vi "fpga_transmission_control_3V14.vi"() -> ()   [LabVIEW 2017]
uses:
  Control 1.ctl
  <vilib>/Platform/TimedLoop/XDataNode/timing_clust.ctl
  <vilib>/Platform/TimedLoop/XDataNode/nitl_modes.ctl
  <vilib>/Platform/TimedLoop/XDataNode/wakeup.ctl
  <vilib>/Instr/_visa.llb/VISA Configure Serial Port (Serial Instr).vi
  <vilib>/platform/TimedLoop/XDataNode/XDataNode.xnode
  <vilib>/Platform/TimedLoop/XDataNode/XDNodeRunTimeDep.lvlib
panel:
  out "Complete Time":u32
  out "Timer":u32
  out "Output":bool
  out "outcome":u32
  out "currentType":string
  out "Time":dbl(slide) scale=0.0..100.0
  out "Progress":dbl(slide) scale=0.0..100.0
  in  "error in (no error)":errorcluster
  out "PWM":bool
  out "pattern":u32
  in  "Timeslot":bool
  out "type":string
  out "Kombi Chart":cluster{u16, i16}(graph)
  out "contingency":string
  in  "Array":T2(array[cluster]) {"duration" step=1}
  out "Timeslot":i32
  out "Sign":bool
  out "deleted portion":u8[](array[numeric])
  out "data":bool
  out "x-y":u16
  out "Error String":string
  out "error out":errorcluster
  out "Int_pixel":i16
  out "Pixel":u16(graph)
  out "AD_Value":i16
  in  "millisecond timer value 2":u32
  out "AD_Chart":i16(graph)
  in  "Path":path
  out "Read":bool
  in  "Stop Program":bool
  in  "Start":bool
  in  "VISA resource name":refnum<visa-resource-name>
  # "UR Elektronik Biologie\nTerminal V 3.8"
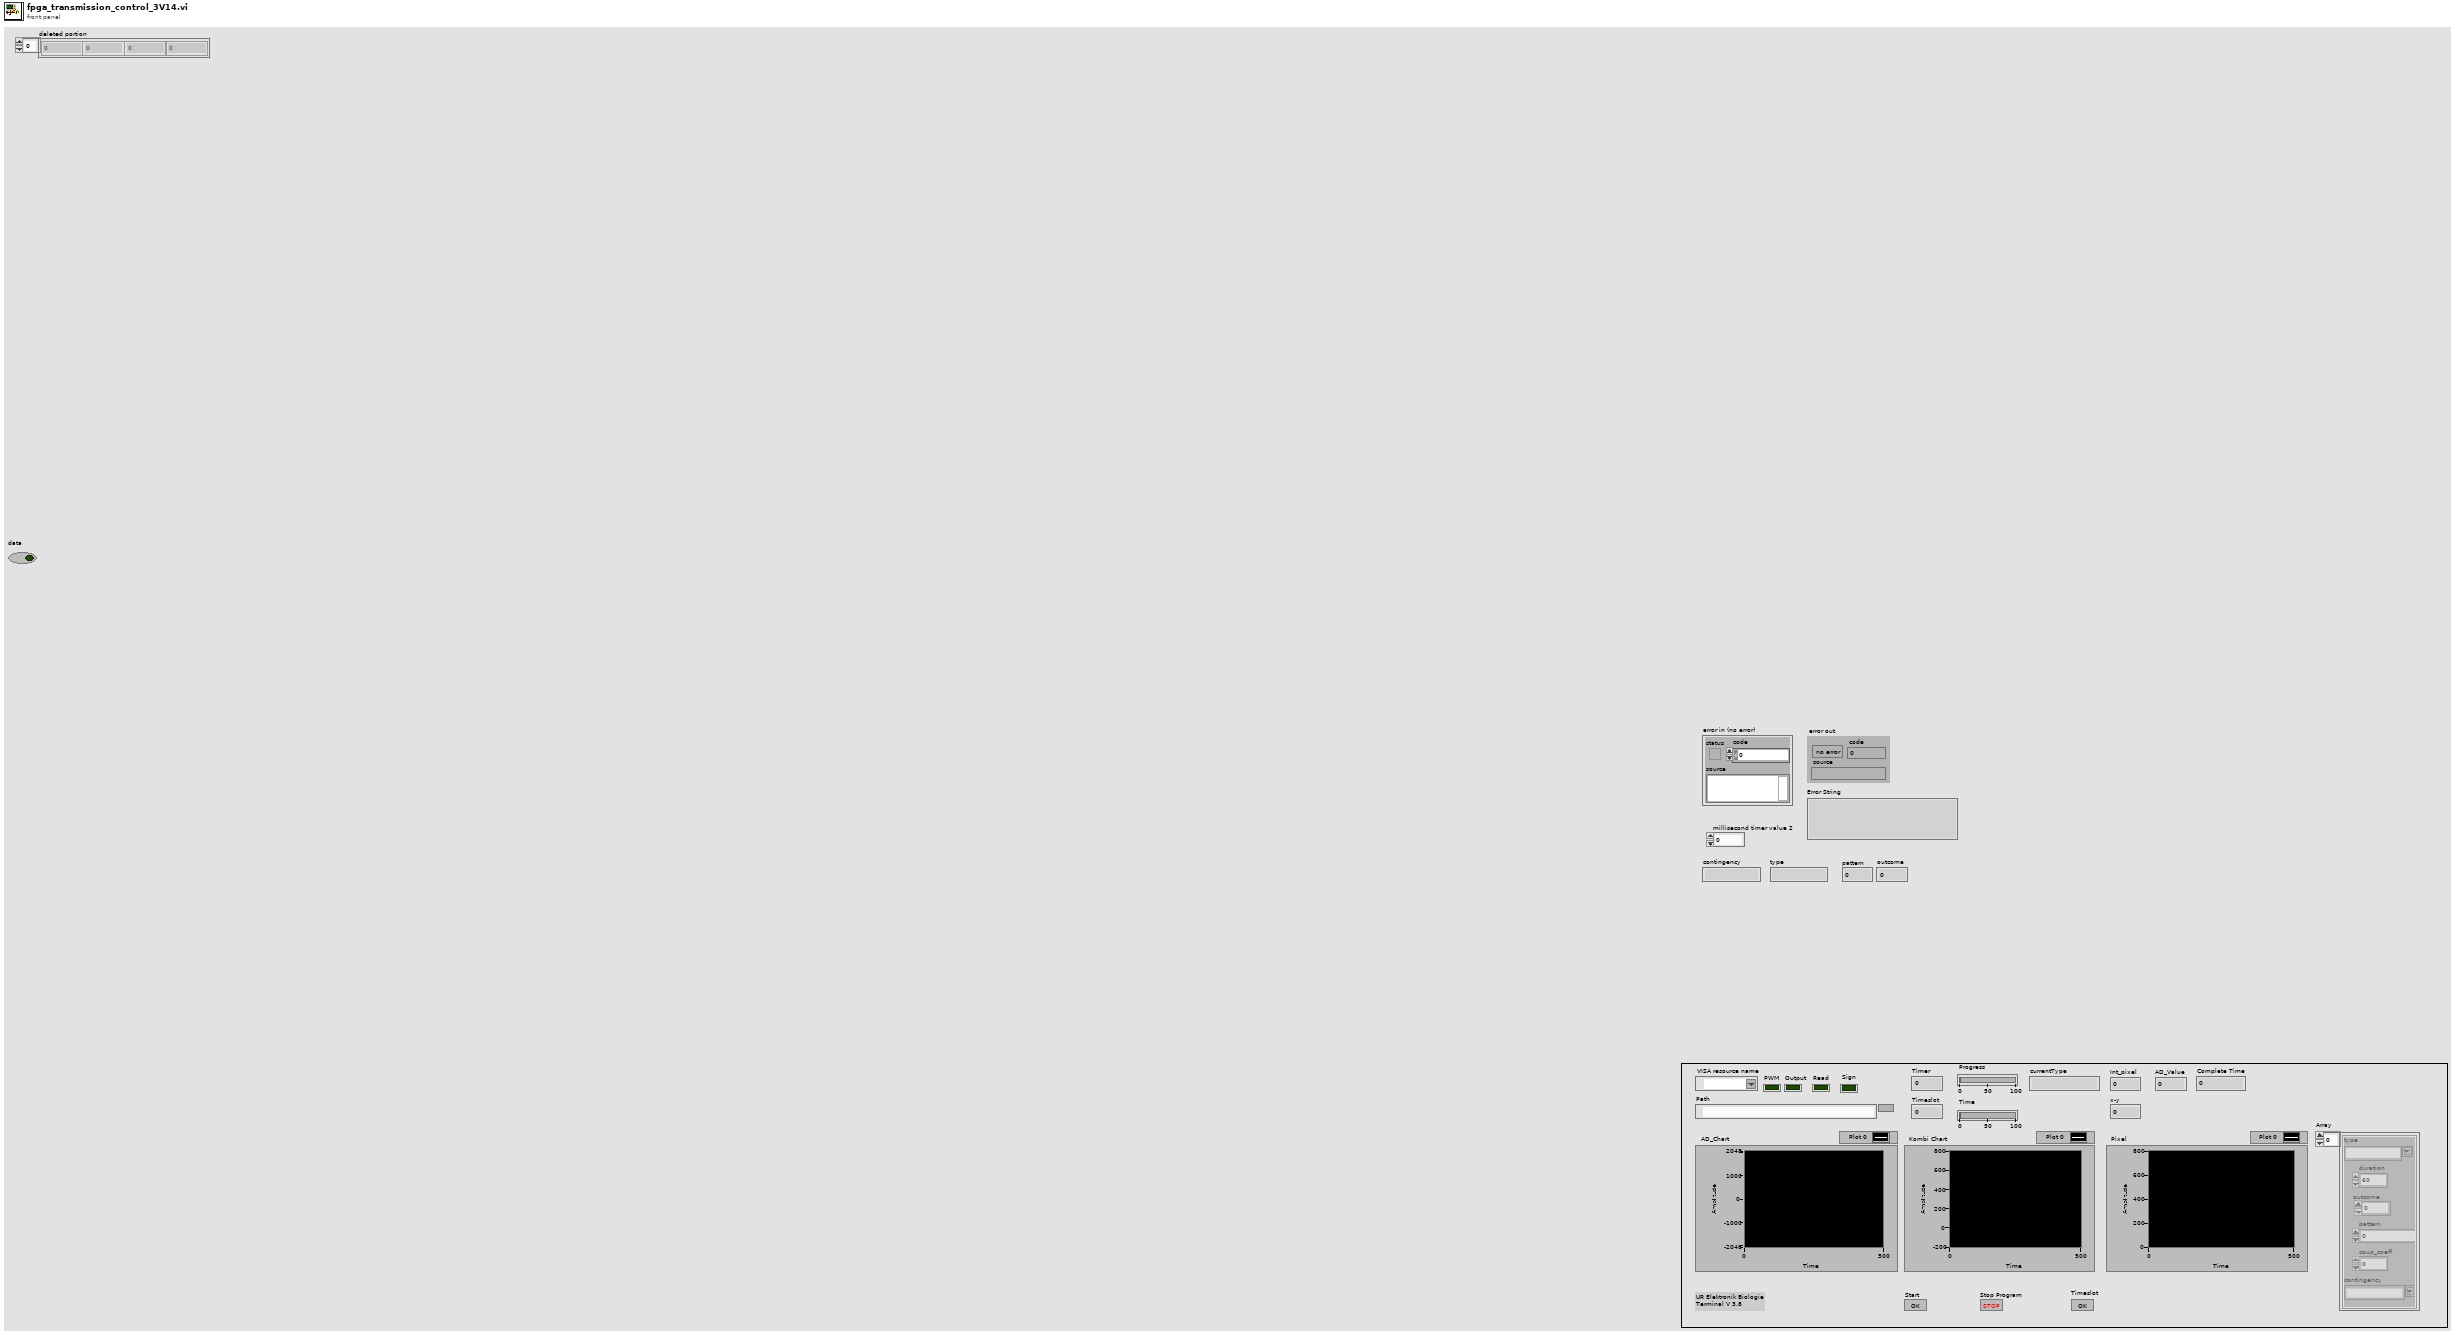
[diagram p1: front panel]
types:
  T1 = typedef "Control 1.ctl" = u32
  T2 = cluster{"type":string, "duration":T1, "outcome":u32, "pattern":u32, "coup_coeff":u32, "contingency":string}[]
  T3 = typedef "XDNodeRunTimeDep.lvlib/timing_clust.ctl" = cluster{"Expected End [f-1]":u64, "Actual End [f-1]":u64, "Finished Late? [f-1]":bool, "Expected End [i-1]":u64, "Actual End [i-1]":u64, "Finished Late? [i-1]":bool, "Expected Start [i]":u64, "Actual Start [i]":u64, "Expected Start [f]":u64, "Actual Start [f]":u64, "Source Name":string, "Structure Name":string, "Period":i64, "Deadline":i64, "Offset":i64, "Start":i64, "Priority":i32, "Timeout":i32, "Mode":T4, "Wakeup Reason":T5, "Error":errorcluster, "Source Type":string, "Secondary Source Type":string, "Global End Time":u64, "Global Start Time":u64, "Frame Duration":u64, "Iteration Duration":u64, "Assigned CPU":i32, "I/O Scan Engine Mode":u32}
  T4 = typedef "XDNodeRunTimeDep.lvlib/nitl_modes.ctl" = enum32{"No Change", "Process missed periods, maintain original phase", "Discard missed periods, maintain original phase", "Process missed periods, ignore original phase", "Discard missed periods, ignore original phase"}
  T5 = typedef "XDNodeRunTimeDep.lvlib/wakeup.ctl" = enum32{"Normal", "Aborted", "Asynchronous wakeup", "Timing source error", "Timed loop error", "Timeout"}
  T6 = cluster{"String":string, i32, i32, u32, u32, "String":string}[]
  T7 = cluster{"type":string, "duration":T1, "outcome":u32, "pattern":u32, "coup_coeff":u32, "contingency":string}
  T8 = enum16{"Idel", "State1", "State2", "State3", "State4"}
  T9 = enum16{"open", "replace", "create", "open or create", "replace or create", "replace or create with confirmation"}
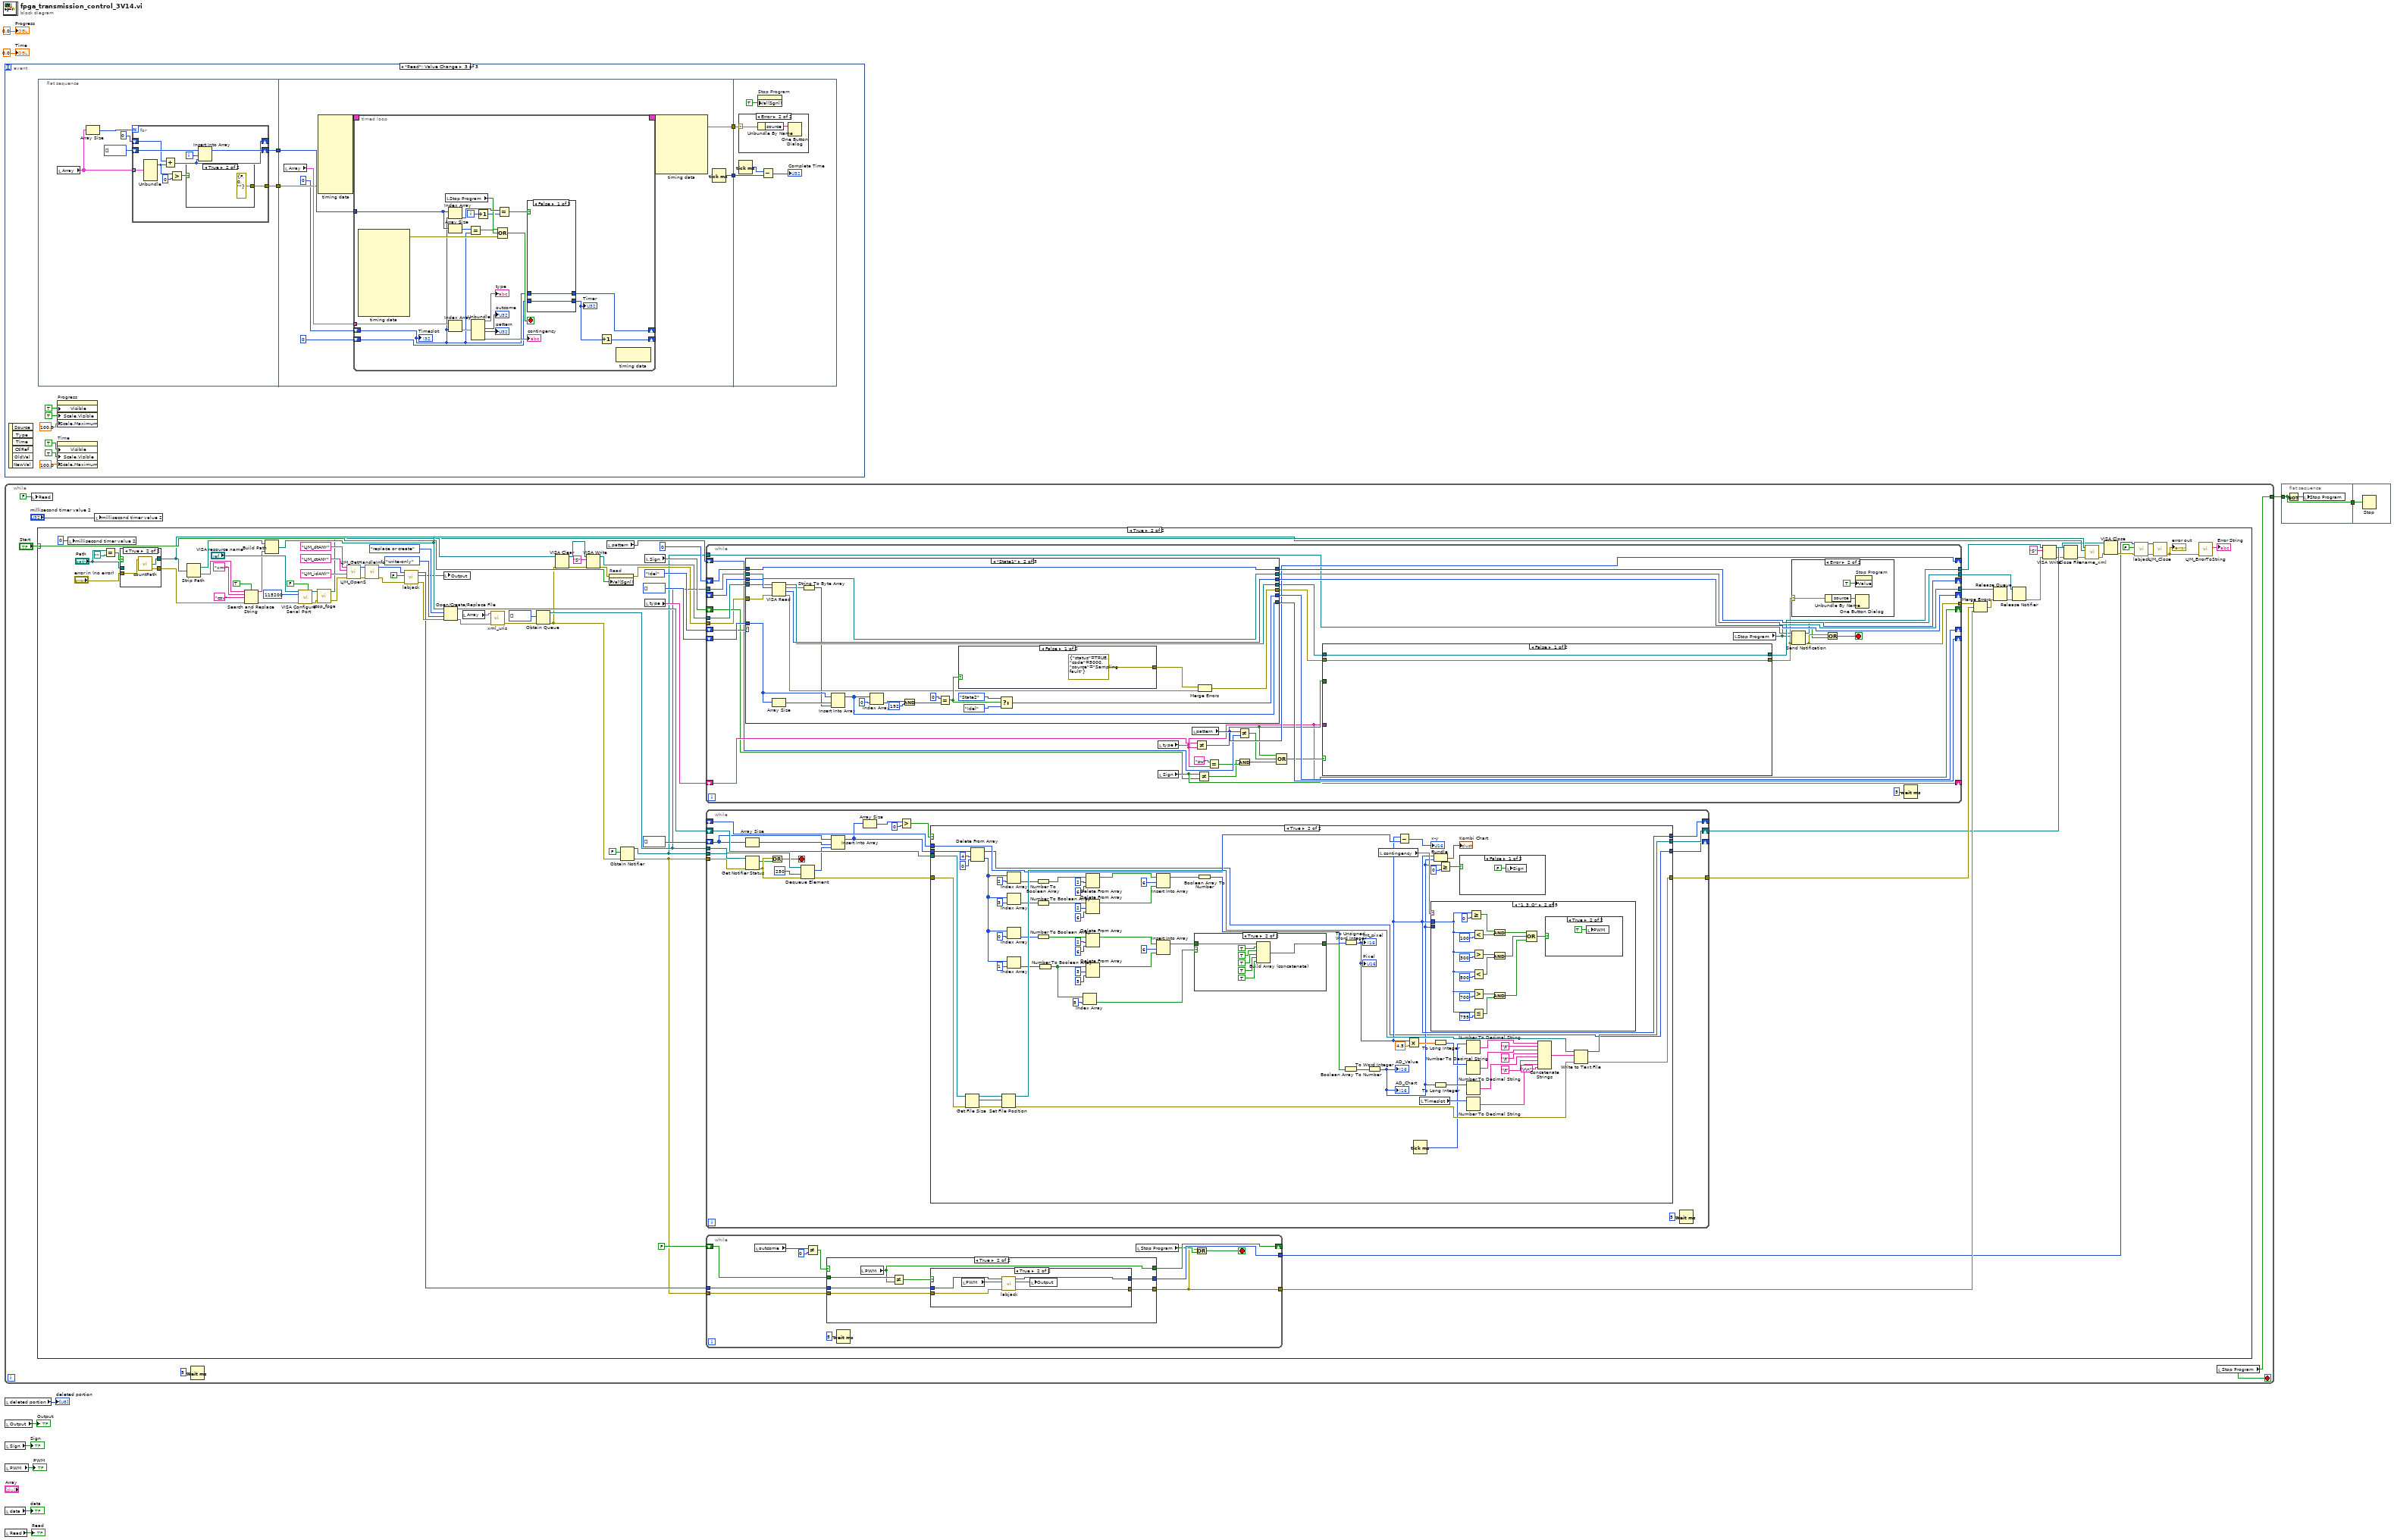
[diagram p0: block diagram]
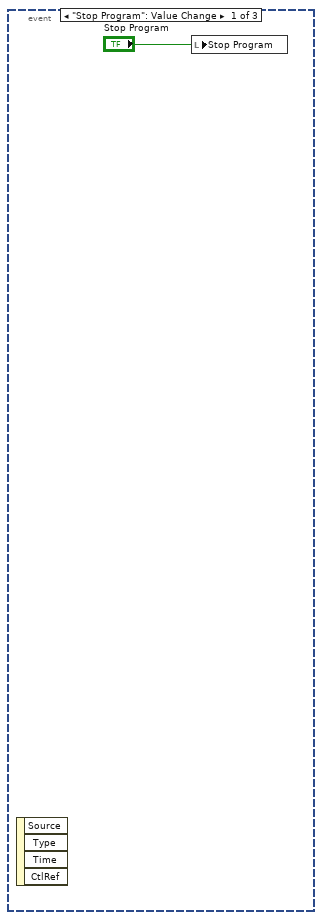
[diagram p2: hidden frame]
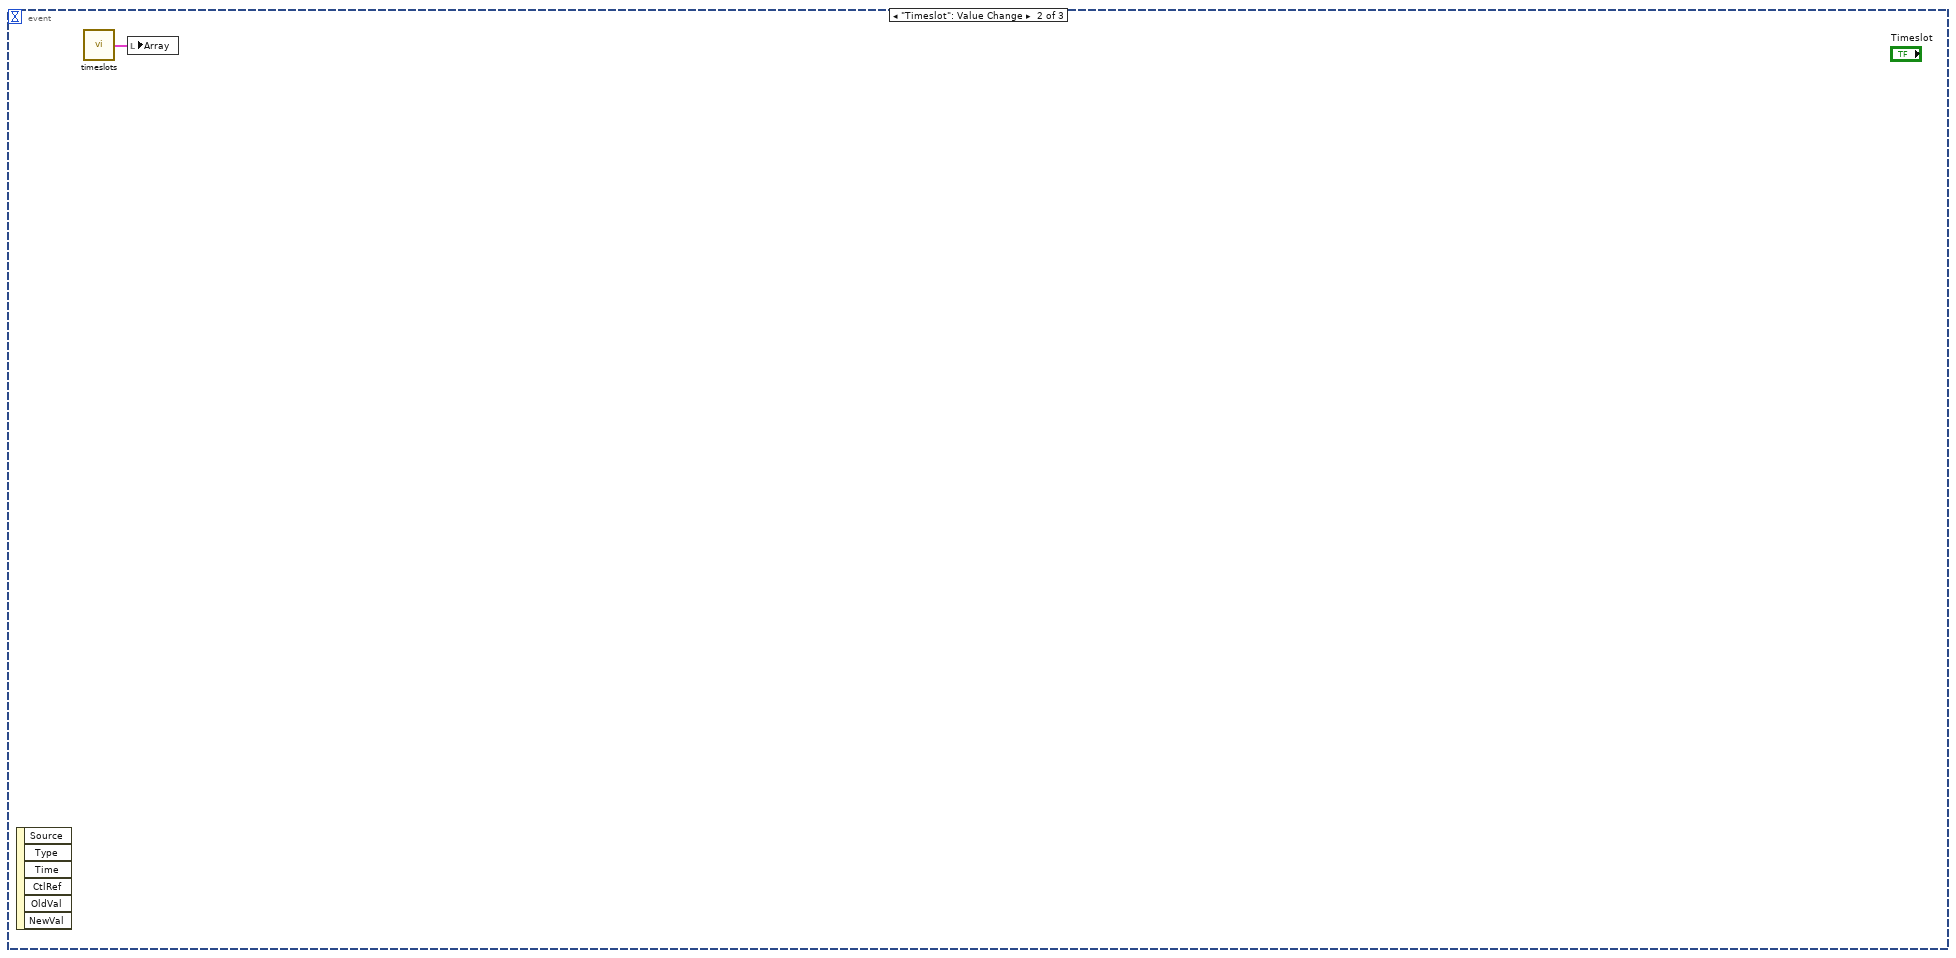
[diagram p3: hidden frame]
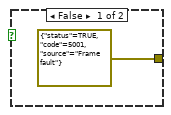
[diagram p4: hidden frame]
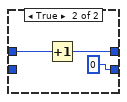
[diagram p5: hidden frame]
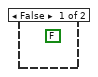
[diagram p7: hidden frame]
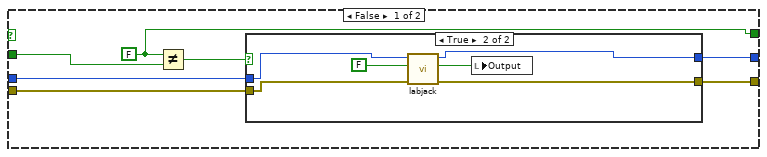
[diagram p9: hidden frame]
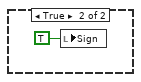
[diagram p13: hidden frame]
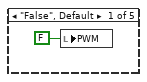
[diagram p14: hidden frame]
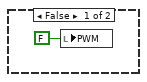
[diagram p15: hidden frame]
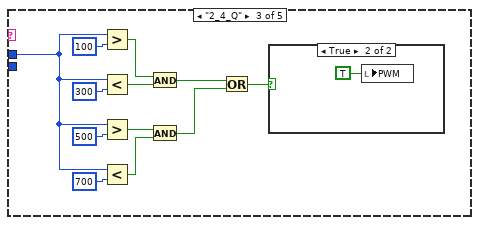
[diagram p16: hidden frame]
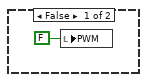
[diagram p17: hidden frame]
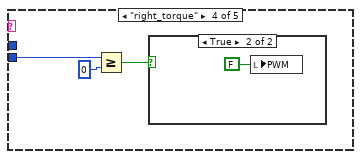
[diagram p18: hidden frame]
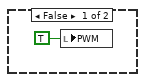
[diagram p19: hidden frame]
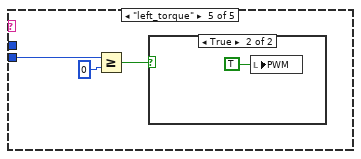
[diagram p20: hidden frame]
diagram:
  n1 = event shown="[2] \"Read\": Value Change" {
    selector: _ -> [_ _ _]
    dyn-events: _ -> [_ _ _]
    timeout: _ -> [_ _ _]
    event "Stop Program": Value Change {
      n2 = event-data() -> ()  [unwired: 1 in, 4 out]
      n3 = local write "Stop Program"("Stop Program") -> ()
    }
    event "Timeslot": Value Change {
      n4 = event-data() -> ()  [unwired: 1 in, 6 out]
      n5 = call "timeslots.vi"() -> ("array of clusters"=w12:T6)  [unwired: 1 in, 1 out]
      n6 = local write "Array"(w12) -> ()
    }
    event "Read": Value Change {
      n7 = event-data() -> ()  [unwired: 1 in, 6 out]
      n8 = flat-sequence {
        tunnel: [w24] -> w16
        tunnel: [w23] -> w15
        tunnel: w16 -> [w46]
        tunnel: w15 -> [w45]
        tunnel: [w44] -> w14
        tunnel: [w42] -> w13
        tunnel: w14 -> [w87]
        tunnel: w13 -> [w84]
        frame #0 {
          n9 = local read "Array"() -> (w27:T2)
          n10 = Array Size(array=w27) -> (size(s)=w28:i32)
          n11 = for {
            N: w28 -> [_]
            tunnel: w27 -> [w38] mode=indexing
            shift-right: [w36] -> w24
            shift-left: T1[] [] -> [w35]
            shift-right: [w33] -> _
            shift-left: T1 0 ("duration") -> [w34]
            tunnel: [w29] -> w23
            i -> [w37]
            n12 = Unbundle(w38) -> ("duration"=w31:T1)  [unwired: 5 out]
            n13 = Add(x=w34, y=w31) -> (x+y=w33:T1)
            n14 = Greater?(x=w31, y=T1 0) -> (0:w32:bool)
            n15 = case shown="True" w32 {
              tunnel: [errorcluster {"status"=TRUE, "code"=5001, "source"="Frame fault"} ("error constant") errorcluster {"status"=FALSE, "code"=0, "source"=""} ("error constant")] -> w29
              frame False {
              }
              frame True {
              }
            }
            n16 = Insert Into Array(array=w35, index=w37, new element=w33) -> (w36:T1[])
          }
        }
        frame #1 {
          n17 = local read "Array"() -> (w47:T2)
          n18 = node-c288(w45) -> (w49:T3)  [unwired: 9 in]
          n19 = timed-loop {
            timing: w49 -> [_]
            timing-out: [_] -> w48
            tunnel: w47 -> [w65]
            tunnel: w46 -> [w59]
            shift-right: [w62] -> _
            shift-left: T1 0 ("duration") -> [w57]
            shift-right: [w52] -> _
            shift-left: 0 -> [w51]
            i -> [w54]
            stop <- w64 stop-if-true
            n20 = node-c288() -> (w63:errorcluster)  [unwired: 1 in, 11 out]
            n21 = local read "Stop Program"() -> (w56:bool)
            n22 = Index Array(array=w59, index=w57) -> (element=w61:T1)
            n23 = Array Size(array=w59) -> (size(s)=w58:i32)
            n24 = Index Array(array=w65, index=w57) -> (element=w70:T7)
            n25 = Equal?(x=w58, y=w57) -> (x = y?=w55:bool)
            n26 = Unbundle(w70) -> ("type"=→"type":string, "outcome"=→"outcome":u32, "pattern"=→"pattern":u32, "contingency"=→"contingency":string)  [unwired: 2 out]
            n27 = Increment(x=w54) -> (x+1=w53:i32)
            n28 = Equal?(x=w61, y=w53) -> (x = y?=w60:bool)
            n29 = Compound Arithmetic op=OR(w56, w55, w63) -> (w64:bool)
            n30 = case shown="False" w60 {
              tunnel: [w72 w75] -> w62
              tunnel: w57 -> [w72 w74]
              tunnel: w51 -> [w71 _]
              tunnel: [w71 0] -> w50
              frame False {
              }
              frame True {
                n31 = Increment(x=w74) -> (x+1=w75:T1)
              }
            }
            "Timer" <- w50
            n32 = Increment(x=w50) -> (x+1=w52:i32)
            n33 = node-c288() -> ()  [unwired: 1 in, 1 out]
            "Timeslot" <- w57
          }
          n34 = node-c288(w48) -> (w44:errorcluster)  [unwired: 6 out]
          n35 = Tick Count (ms)() -> (millisecond timer value=w42:u32)
        }
        frame #2 {
          n36 = case shown="Error" w87 {
            selector: w87 -> [_ w90]
            frame No Error {
            }
            frame Error {
              n37 = Unbundle By Name(w90) -> ("source"=w89:string)
              n38 = One Button Dialog(message=w89) -> ()  [unwired: 1 in, 1 out]
            }
          }
          n39 = Tick Count (ms)() -> (millisecond timer value=w85:u32)
          n40 = property on="Stop Program" class="Bool (strict)"("Val(Sgnl)"=TRUE) -> ()  [unwired: 2 in, 2 out]
          n41 = Subtract(x=w85, y=w84) -> (x-y=→"Complete Time":u32)
        }
      }
      n42 = property on="Progress" class="Slide (strict)"("Visible"=TRUE, "Scale.Visible"=TRUE ("Visible"), "Scale.Maximum"=100.0 ("Scale.Range:Maximum")) -> ()  [unwired: 2 in, 2 out]
      n43 = property on="Time" class="Slide (strict)"("Visible"=TRUE, "Scale.Visible"=TRUE ("Visible"), "Scale.Maximum"=100.0 ("Scale.Range:Maximum")) -> ()  [unwired: 2 in, 2 out]
    }
  }
  n44 = while {
    tunnel: [w94] -> w10
    stop <- w94 stop-if-true
    n45 = local write "Read"(FALSE) -> ()
    n46 = case shown="True" "Start" {
      selector: "Start" -> [_ w171]
      frame False {
        (unwired) FALSE
      }
      frame True {
        n47 = local write "millisecond timer value 2"(u32 0 ("millisecond timer value 2")) -> ()
        n48 = Equal?(x="Path", y=path "") -> (x = y?=w159:bool)
        n49 = case shown="True" w159 {
          tunnel: [w179 w182] -> w125
          tunnel: "Path" -> [w179 _]
          tunnel: [w178 w181] -> w134
          tunnel: "error in (no error)" -> [w178 w180]
          frame False {
          }
          frame True {
            n50 = call "countPath.vi"("error in (no error)"=w180) -> ("error out"=w181:errorcluster, "appended path"=w182:path)
          }
        }
        n51 = Strip Path(path=w125) -> (stripped path=w138:path, name=w137:string)
        n52 = Search and Replace String(case sensitive?=TRUE ("ignore case? (F)"), input string=w137, search string="xml", replace string="csv" ("replace string (\"\")"), error in=w134) -> (result string=w131:string, error out=w133:errorcluster)  [unwired: 3 in, 2 out]
        n53 = Build Path(base path=w138, name or relative path=w131) -> (appended path=w126:path)
        n54 = call-poly "VISA Configure Serial Port"("VISA resource name"="VISA resource name", "Enable Termination\nChar (T)"=FALSE ("Enable Termination\nChar (T)"), "baud rate (9600)"=u32 115200, "error in (no error)"=w133) -> ("VISA resource name out"=w118:refnum<visa-resource-name>, "error out"=w117:errorcluster)  [unwired: 10 in]
        n55 = call "stop_fpga.vi"("error in (no error)"=w117, "reference"=w118) -> ("error out"=w116:errorcluster, "VISA resource name out"=w109:refnum<visa-resource-name>)  [unwired: 2 in]
        n56 = call "LJM_OpenS.vi"("error in"=w116, "Identifier"="LJM_idANY", "ConnectionType"="LJM_ctANY", "DeviceType"="LJM_dtANY") -> ("error out"=w162:errorcluster, "Handle"=w161:i32)  [unwired: 6 in]
        n57 = call "LJM_GetHandleInfo.vi"("error in"=w162, "Handle In"=w161) -> ("error out"=w164:errorcluster, "Handle Out"=w163:i32)  [unwired: 2 in, 6 out]
        n58 = call "labjack.vi"("error out"=w164, "Boolean"=FALSE, "Handle Out"=w163) -> ("error out 2"=w167:errorcluster, "Boolean 2"=w124:bool, "Handle Out 2"=w166:i32)  [unwired: 6 in]
        n59 = local write "Output"(w124) -> ()
        n60 = Open/Create/Replace File(file path (use dialog)=w126, error in=w167, operation (0:open)=T9."replace or create", access (0:read/write)=enum16{"read/write", "read-only", "write-only"}."write-only") -> (refnum out=w141:refnum<file>, error out=w139:errorcluster)  [unwired: 2 in, 1 out]
        n61 = local read "Array"() -> (w140:T2)
        n62 = call "xml_uris.vi"("error in"=w139, "Array"=w140) -> ("error out"=w110:errorcluster)  [unwired: 2 in, 2 out]
        n63 = Obtain Queue(element data type=u8[] [], error in (no error)=w110) -> (queue out=w112:refnum<queue>, error out=w97:errorcluster)  [unwired: 3 in, 1 out]
        n64 = VISA Clear(VISA resource name=w109, error in (no error)=w97) -> (VISA resource name out=w108:refnum<visa-resource-name>, error out=w106:errorcluster)
        n65 = VISA Write(VISA resource name=w108, write buffer="S", error in (no error)=w106) -> (VISA resource name out=w107:refnum<visa-resource-name>, error out=w115:errorcluster)  [unwired: 1 out]
        n66 = local read "pattern"() -> (w144:u32)
        n67 = property on="Read" class="Bool (strict)"(error in=w115, "Val(Sgnl)"=w171) -> (error out=w105:errorcluster)  [unwired: 1 in, 1 out]
        n68 = Obtain Notifier(notification data type=FALSE, error in (no error)=w97) -> (notifier out=w103:refnum<notifier>, error out=w96:errorcluster)  [unwired: 2 in, 1 out]
        n69 = local read "Sign"() -> (w143:bool)
        n70 = local read "type"() -> (w168:string)
        n71 = while {
          tunnel: w107 -> [w409]
          shift-right: [w403] -> _
          shift-left: u8[] [] -> [w408]
          tunnel: [w385] -> w121
          shift-right: [w407] -> _
          shift-left: T8."Idel" -> [w406]
          shift-right: [w405] -> _
          shift-left: _ -> [w404]
          shift-right: [w402] -> _
          shift-left: u8 0 -> [w401]
          shift-right: [w392] -> _
          shift-left: w168 -> [w400]
          shift-right: [w399] -> _
          shift-left: w144 -> [w398]
          shift-right: [w397] -> _
          shift-left: w143 -> [w396]
          tunnel: w112 -> [w384]
          tunnel: [w383] -> w111
          tunnel: w103 -> [w380]
          tunnel: w105 -> [w381]
          tunnel: [w377] -> w100
          tunnel: [w378] -> w101
          stop <- w375 stop-if-true
          n72 = case shown="\"State1\"" w406 {
            tunnel: w409 -> [w527 w554 w572]
            tunnel: w381 -> [w528 w555 w566]
            tunnel: w408 -> [w531 w557 w579]
            tunnel: [w535 w558 w572] -> w386
            tunnel: [w534 w543 w565] -> w387
            tunnel: [w536 w556 w575] -> w407
            tunnel: [w533 w559 w573] -> w405
            tunnel: w404 -> [_ w560 w573]
            tunnel: [w531 w553 w578] -> w403
            tunnel: [w530 w552 u8 0] -> w402
            tunnel: w401 -> [w530 w552 _]
            tunnel: w384 -> [w525 w546 w568]
            tunnel: [w525 w546 w567] -> w383
            frame "Idel", Default {
              n73 = local write "data"(FALSE ("data")) -> ()
              n74 = property class="Serial Instr"(reference=w527, error in=w528) -> (reference out=w535:refnum<visa-resource-name>, error out=w534:errorcluster, "Serial Settings:Number of Bytes at Serial Port"=w533:u32)
              n75 = Greater Or Equal?(x=w533, y=u8 4) -> (x >= y?=w526:bool)
              n76 = Select(t=T8."State1", s=w526, f=T8."Idel") -> (s? t:f=w536:T8)
            }
            frame "State1" {
              n77 = VISA Read(VISA resource name=w554, byte count=w560, error in (no error)=w555) -> (VISA resource name out=w558:refnum<visa-resource-name>, read buffer=w540:string, return count=w559:u32, error out=w541:errorcluster)
              n78 = Array Size(array=w557) -> (size(s)=w545:i32)
              n79 = String To Byte Array(string=w540) -> (unsigned byte array=w539:u8[])
              n80 = Insert Into Array(array=w557, index=w545, new element=w539) -> (w553:u8[])
              n81 = Index Array(array=w553, index=0) -> (element=w550:u8)
              n82 = And(x=w550, y=u8 192) -> (x .and. y?=w549:u8)
              n83 = Equal?(x=u8 0, y=w549) -> (x = y?=w542:bool)
              n84 = case shown="False" w542 {
                tunnel: [errorcluster {"status"=TRUE, "code"=5000, "source"="Sampling fault"} ("error constant") errorcluster {"status"=FALSE, "code"=0, "source"=""} ("error constant")] -> w544
                frame False {
                }
                frame True {
                }
              }
              n85 = Select(t=T8."State2", s=w542, f=T8."Idel") -> (s? t:f=w556:T8)
              n86 = Merge Errors(w544, w541) -> (w543:errorcluster)
            }
            frame "State2" {
              n87 = Delete From Array(array=w579, length=4, index=0) -> (deleted portion=w569:u8[], array with subset deleted=w578:u8[])
              n88 = Array Size(array=w578) -> (size(s)=w577:i32)
              n89 = Enqueue Element(queue=w568, element=w569, error in (no error)=w566) -> (queue out=w567:refnum<queue>, error out=w565:errorcluster)  [unwired: 1 in, 1 out]
              n90 = Greater Or Equal?(x=w577, y=4) -> (x >= y?=w570:bool)
              n91 = Select(t=T8."State2", s=w570, f=T8."Idel") -> (s? t:f=w575:T8)
            }
          }
          n92 = local read "type"() -> (w392:string)
          n93 = local read "Sign"() -> (w397:bool)
          n94 = local read "pattern"() -> (w399:u32)
          n95 = Not Equal?(x=w400, y=w392) -> (x != y?=w393:bool)
          n96 = Not Equal?(x=w397, y=w396) -> (x != y?=w389:bool)
          n97 = Equal?(x="sw", y=w392) -> (x = y?=w390:bool)
          n98 = Not Equal?(x=w399, y=w398) -> (x != y?=w395:bool)
          n99 = And(x=w389, y=w390) -> (x .and. y?=w388:bool)
          n100 = Compound Arithmetic op=OR(w393, w395, w388) -> (w394:bool)
          n101 = case shown="False" w394 {
            tunnel: w386 -> [w414 w418]
            tunnel: [w414 w421] -> w385
            tunnel: w387 -> [w413 w417]
            tunnel: [w413 w422] -> w379
            tunnel: w392 -> [_ w415]
            tunnel: w393 -> [_ w416]
            frame False {
            }
            frame True {
              n102 = case shown="True" w416 {
                tunnel: [w424 w430] -> w420
                tunnel: [w425 w429] -> w419
                tunnel: w418 -> [w425 w427]
                tunnel: w417 -> [w424 w426]
                frame False {
                }
                frame True {
                  n103 = VISA Write(VISA resource name=w427, write buffer="1W", error in (no error)=w426) -> (VISA resource name out=w429:refnum<visa-resource-name>, error out=w430:errorcluster)  [unwired: 1 out]
                }
              }
              n104 = case shown="\"fs\"" w415 {
                tunnel: w419 -> [w432 w439 w444 w452 w463 w500]
                tunnel: [w434 w438 w443 w446 w462 w499] -> w421
                tunnel: w420 -> [w431 w437 w442 w451 w465 w502]
                tunnel: [w433 w436 w441 w447 w464 w501] -> w423
                frame "False", Default {
                  n105 = VISA Write(VISA resource name=w432, write buffer="s4s", error in (no error)=w431) -> (VISA resource name out=w434:refnum<visa-resource-name>, error out=w433:errorcluster)  [unwired: 1 out]
                }
                frame "optomotorR" {
                  n106 = VISA Write(VISA resource name=w439, write buffer="s3r", error in (no error)=w437) -> (VISA resource name out=w438:refnum<visa-resource-name>, error out=w436:errorcluster)  [unwired: 1 out]
                }
                frame "optomotorL" {
                  n107 = VISA Write(VISA resource name=w444, write buffer="s3l", error in (no error)=w442) -> (VISA resource name out=w443:refnum<visa-resource-name>, error out=w441:errorcluster)  [unwired: 1 out]
                }
                frame "yt" {
                  n108 = local read "pattern"() -> (w450:u32)
                  n109 = VISA Write(VISA resource name=w452, write buffer="s1s", error in (no error)=w451) -> (VISA resource name out=w449:refnum<visa-resource-name>, error out=w448:errorcluster)  [unwired: 1 out]
                  n110 = case shown="9" w450 {
                    tunnel: w449 -> [w455 w459]
                    tunnel: w448 -> [w454 w458]
                    tunnel: [w454 w457] -> w447
                    tunnel: [w455 w456] -> w446
                    frame 0, Default {
                    }
                    frame 9 {
                      n111 = VISA Write(VISA resource name=w459, write buffer="D", error in (no error)=w458) -> (VISA resource name out=w456:refnum<visa-resource-name>, error out=w457:errorcluster)  [unwired: 1 out]
                    }
                  }
                }
                frame "sw" {
                  n112 = local read "pattern"() -> (w461:u32)
                  n113 = case shown="7" w461 {
                    tunnel: w465 -> [w466 w471 w487]
                    tunnel: [w466 w469 w486] -> w464
                    tunnel: w463 -> [w467 w472 w485]
                    tunnel: [w467 w470 w484] -> w462
                    frame 0, Default {
                    }
                    frame 8 {
                      n114 = local read "Sign"() -> (w468:bool)
                      n115 = case shown="False" w468 {
                        tunnel: w471 -> [w474 w481]
                        tunnel: [w473 w480] -> w469
                        tunnel: w472 -> [w476 w479]
                        tunnel: [w475 w478] -> w470
                        frame True {
                          n116 = VISA Write(VISA resource name=w476, write buffer="G", error in (no error)=w474) -> (VISA resource name out=w475:refnum<visa-resource-name>, error out=w473:errorcluster)  [unwired: 1 out]
                        }
                        frame False {
                          n117 = VISA Write(VISA resource name=w479, write buffer="B", error in (no error)=w481) -> (VISA resource name out=w478:refnum<visa-resource-name>, error out=w480:errorcluster)  [unwired: 1 out]
                        }
                      }
                    }
                    frame 7 {
                      n118 = local read "Sign"() -> (w483:bool)
                      n119 = case shown="True" w483 {
                        tunnel: w487 -> [w489 w496]
                        tunnel: [w488 w495] -> w486
                        tunnel: w485 -> [w491 w494]
                        tunnel: [w490 w493] -> w484
                        frame False {
                          n120 = VISA Write(VISA resource name=w491, write buffer="G", error in (no error)=w489) -> (VISA resource name out=w490:refnum<visa-resource-name>, error out=w488:errorcluster)  [unwired: 1 out]
                        }
                        frame True {
                          n121 = VISA Write(VISA resource name=w494, write buffer="B", error in (no error)=w496) -> (VISA resource name out=w493:refnum<visa-resource-name>, error out=w495:errorcluster)  [unwired: 1 out]
                        }
                      }
                    }
                  }
                }
                frame "fs" {
                  n122 = local read "pattern"() -> (w498:u32)
                  n123 = case shown="4" w498 {
                    tunnel: w502 -> [w503 w509 w514 w519 w524]
                    tunnel: [w503 w507 w512 w517 w522] -> w501
                    tunnel: w500 -> [w504 w508 w513 w518 w523]
                    tunnel: [w504 w506 w511 w516 w521] -> w499
                    frame 0, Default {
                    }
                    frame 3 {
                      n124 = VISA Write(VISA resource name=w508, write buffer="s3s", error in (no error)=w509) -> (VISA resource name out=w506:refnum<visa-resource-name>, error out=w507:errorcluster)  [unwired: 1 out]
                    }
                    frame 2 {
                      n125 = VISA Write(VISA resource name=w513, write buffer="s2s", error in (no error)=w514) -> (VISA resource name out=w511:refnum<visa-resource-name>, error out=w512:errorcluster)  [unwired: 1 out]
                    }
                    frame 1 {
                      n126 = VISA Write(VISA resource name=w518, write buffer="s1s", error in (no error)=w519) -> (VISA resource name out=w516:refnum<visa-resource-name>, error out=w517:errorcluster)  [unwired: 1 out]
                    }
                    frame 4 {
                      n127 = VISA Write(VISA resource name=w523, write buffer="s4s", error in (no error)=w524) -> (VISA resource name out=w521:refnum<visa-resource-name>, error out=w522:errorcluster)  [unwired: 1 out]
                    }
                  }
                }
              }
              n128 = feedback #1() -> (w422:errorcluster)  [unwired: 1 in]
              n129 = feedback-in #1(w423) -> ()
              "currentType" <- w415
            }
          }
          n130 = local read "Stop Program"() -> (w376:bool)
          n131 = case shown="Error" w379 {
            selector: w379 -> [_ w411]
            frame No Error {
            }
            frame Error {
              n132 = Unbundle By Name(w411) -> ("source"=w410:string)
              n133 = property on="Stop Program" class="Bool (strict)"("Value"=TRUE) -> ()  [unwired: 2 in, 2 out]
              n134 = One Button Dialog(message=w410) -> ()  [unwired: 1 in, 1 out]
            }
          }
          n135 = Send Notification(notification=w376, notifier=w380, error in (no error)=w379) -> (notifier out=w378:refnum<notifier>, error out=w377:errorcluster)
          n136 = Or(x=w377, y=w376) -> (x .or. y?=w375:bool)
          n137 = Wait (ms)(milliseconds to wait=u32 5) -> ()  [unwired: 1 out]
        }
        n138 = while {
          shift-right: [w245] -> w129
          shift-left: w141 -> [w246]
          shift-right: [w243] -> _
          shift-left: _ -> [w244]
          shift-right: [w239] -> _
          shift-left: u8[] [] -> [w240]
          tunnel: w112 -> [w228]
          tunnel: w103 -> [w231]
          tunnel: w96 -> [w230]
          tunnel: [w242] -> w130
          stop <- w227 stop-if-true
          n139 = Array Size(array=w240) -> (size(s)=w238:i32)
          n140 = Get Notifier Status(notifier=w231, error in (no error)=w230) -> (current notification=w225:bool, error out=w226:errorcluster)  [unwired: 3 out]
          n141 = Or(x=w226, y=w225) -> (x .or. y?=w227:bool)
          n142 = Dequeue Element(queue=w228, timeout in ms (-1)=250, error in (no error)=w226) -> (element=w235:u8[], error out=w232:errorcluster)  [unwired: 2 out]
          n143 = Insert Into Array(array=w240, index=w238, new element=w235) -> (w234:u8[])
          n144 = Array Size(array=w234) -> (size(s)=w233:i32)
          n145 = Greater?(x=w233, y=0) -> (0:w236:bool)
          n146 = case shown="True" w236 {
            tunnel: w232 -> [w250 w272]
            tunnel: [w250 w315] -> w242
            tunnel: w246 -> [w249 w278]
            tunnel: [w249 w314] -> w245
            tunnel: [w248 w258] -> w243
            tunnel: w244 -> [w248 w273]
            tunnel: w234 -> [w247 w256]
            tunnel: [w247 w253] -> w239
            frame False {
            }
            frame True {
              n147 = Get File Size(file=w278, error in=w272) -> (refnum out=w320:refnum<file>, size (in bytes)=w319:i64, 0:w318:errorcluster)
              n148 = Delete From Array(array=w256, length=4, index=0) -> (deleted portion=w252:u8[], array with subset deleted=w253:u8[])
              n149 = Set File Position(offset (in bytes) (0)=w319, refnum=w320, error in=w318) -> (refnum out=w316:refnum<file>, error out=w317:errorcluster)  [unwired: 1 in]
              n150 = Index Array(array=w252, index=2) -> (element=w275:u8)
              n151 = Index Array(array=w252, index=3) -> (element=w274:u8)
              n152 = Index Array(array=w252, index=0) -> (element=w277:u8)
              n153 = Index Array(array=w252, index=1) -> (element=w276:u8)
              n154 = Number To Boolean Array(number=w275) -> (Boolean array=w296:bool[])
              n155 = Number To Boolean Array(number=w274) -> (Boolean array=w299:bool[])
              n156 = Number To Boolean Array(number=w277) -> (Boolean array=w286:bool[])
              n157 = Number To Boolean Array(number=w276) -> (Boolean array=w305:bool[])
              n158 = Index Array(array=w305, index=5) -> (element=w307:bool)
              n159 = Delete From Array(array=w296, length=2, index=6 ("length")) -> (array with subset deleted=w309:bool[])  [unwired: 1 out]
              n160 = Delete From Array(array=w299, length=2, index=6) -> (array with subset deleted=w310:bool[])  [unwired: 1 out]
              n161 = Delete From Array(array=w286, length=2, index=6 ("length")) -> (array with subset deleted=w289:bool[])  [unwired: 1 out]
              n162 = Delete From Array(array=w305, length=3, index=5) -> (array with subset deleted=w294:bool[])  [unwired: 1 out]
              n163 = Insert Into Array(array=w309, index=6, new element=w310) -> (w303:bool[])
              n164 = Insert Into Array(array=w289, index=6, new element=w294) -> (w291:bool[])
              n165 = case shown="True" w307 {
                tunnel: w291 -> [w367 w374]
                tunnel: [w367 w369] -> w308
                frame False {
                }
                frame True {
                  n166 = Build Array (concatenate)(w374, TRUE ("new element/subarray"), TRUE ("new element/subarray"), TRUE ("new element/subarray"), TRUE ("new element/subarray"), TRUE ("element")) -> (w369:bool[])
                }
              }
              n167 = Boolean Array To Number(Boolean array=w303) -> (number=w304:u32)
              n168 = To Unsigned Word Integer(number=w304) -> (unsigned 16bit integer=w258:u16)
              "Pixel" <- w258
              "Int_pixel" <- w258
              n169 = Boolean Array To Number(Boolean array=w308) -> (number=w295:u32)
              n170 = To Word Integer(number=w295) -> (16bit integer=w257:i16)
              "AD_Chart" <- w257
              "AD_Value" <- w257
              n171 = local read "contingency"() -> (w262:string)
              n172 = Subtract(x=w258, y=w273) -> (x-y=→"x-y":u16)
              n173 = Multiply(x=w258, y=4.5) -> (x*y=w264:dbl)
              n174 = Tick Count (ms)() -> (millisecond timer value=w251:u32)
              n175 = local read "Timeslot"() -> (w268:i32)
              n176 = case shown="\"1_3_Q\"" w262 {
                tunnel: w258 -> [_ w325 w351 _ _]
                tunnel: w257 -> [_ _ _ w357 w362]
                frame "False", Default {
                  n177 = local write "PWM"(FALSE ("pwm")) -> ()
                }
                frame "1_3_Q" {
                  n178 = Greater Or Equal?(x=w325, y=u16 0 ("x")) -> (x >= y?=w324:bool)
                  n179 = Less?(x=w325, y=u16 100) -> (x < y?=w335:bool)
                  n180 = Greater?(x=w325, y=u16 300 ("a")) -> (0:w337:bool)
                  n181 = Less?(x=w325, y=u16 500 ("b")) -> (x < y?=w336:bool)
                  n182 = Greater?(x=w325, y=u16 700) -> (0:w334:bool)
                  n183 = Less Or Equal?(x=w325, y=u16 799) -> (x <= y?=w332:bool)
                  n184 = And(x=w324, y=w335) -> (x .and. y?=w330:bool)
                  n185 = And(x=w337, y=w336) -> (x .and. y?=w329:bool)
                  n186 = And(x=w334, y=w332) -> (x .and. y?=w328:bool)
                  n187 = Compound Arithmetic op=OR(w330, w329, w328) -> (w327:bool)
                  n188 = case shown="True" w327 {
                    frame False {
                      n189 = local write "PWM"(FALSE ("pwm")) -> ()
                    }
                    frame True {
                      n190 = local write "PWM"(TRUE ("pwm")) -> ()
                    }
                  }
                }
                frame "2_4_Q" {
                  n191 = Greater?(x=w351, y=u16 100 ("x")) -> (0:w346:bool)
                  n192 = Less?(x=w351, y=u16 300) -> (x < y?=w347:bool)
                  n193 = Greater?(x=w351, y=u16 500 ("a")) -> (0:w350:bool)
                  n194 = Less?(x=w351, y=u16 700 ("b")) -> (x < y?=w348:bool)
                  n195 = And(x=w346, y=w347) -> (x .and. y?=w345:bool)
                  n196 = And(x=w350, y=w348) -> (x .and. y?=w349:bool)
                  n197 = Or(x=w345, y=w349) -> (x .or. y?=w344:bool)
                  n198 = case shown="True" w344 {
                    frame False {
                      n199 = local write "PWM"(FALSE ("pwm")) -> ()
                    }
                    frame True {
                      n200 = local write "PWM"(TRUE ("pwm")) -> ()
                    }
                  }
                }
                frame "right_torque" {
                  n201 = Greater Or Equal?(x=w357, y=i16 0) -> (x >= y?=w358:bool)
                  n202 = case shown="True" w358 {
                    frame False {
                      n203 = local write "PWM"(TRUE ("pwm")) -> ()
                    }
                    frame True {
                      n204 = local write "PWM"(FALSE ("pwm")) -> ()
                    }
                  }
                }
                frame "left_torque" {
                  n205 = Greater Or Equal?(x=w362, y=i16 0) -> (x >= y?=w363:bool)
                  n206 = case shown="True" w363 {
                    frame False {
                      n207 = local write "PWM"(FALSE ("pwm")) -> ()
                    }
                    frame True {
                      n208 = local write "PWM"(TRUE ("pwm")) -> ()
                    }
                  }
                }
              }
              n209 = To Long Integer(number=w264) -> (32bit integer=w263:i32)
              n210 = To Long Integer(number=w257) -> (32bit integer=w266:i32)
              n211 = Bundle(w258, w257) -> (→"Kombi Chart":cluster{u16, i16})  [unwired: 1 in]
              n212 = Greater Or Equal?(x=w257, y=i16 0) -> (x >= y?=w259:bool)
              n213 = case shown="False" w259 {
                frame False {
                  n214 = local write "Sign"(FALSE) -> ()
                }
                frame True {
                  n215 = local write "Sign"(TRUE) -> ()
                }
              }
              n216 = Number To Decimal String(number=w251) -> (decimal integer string=w271:string)  [unwired: 1 in]
              n217 = Number To Decimal String(number=w263) -> (decimal integer string=w311:string)  [unwired: 1 in]
              n218 = Number To Decimal String(number=w266) -> (decimal integer string=w269:string)  [unwired: 1 in]
              n219 = Number To Decimal String(number=w268) -> (decimal integer string=w267:string)  [unwired: 1 in]
              n220 = Concatenate Strings(w271, "\t" ("string"), w311, "\t" ("string"), w269, "\t" ("string"), w267, "\r\n") -> (w279:string)
              n221 = Write to Text File(file (use dialog)=w316, text=w279, error in=w317) -> (refnum out=w314:refnum<file>, error out=w315:errorcluster)  [unwired: 1 in, 1 out]
            }
          }
          n222 = Wait (ms)(milliseconds to wait=u32 5) -> ()  [unwired: 1 out]
        }
        n223 = while {
          tunnel: w166 -> [w193]
          tunnel: w96 -> [w192]
          shift-right: [w190] -> _
          shift-left: FALSE ("pwm") -> [w194]
          tunnel: [w191] -> w148
          tunnel: [w183] -> w172
          stop <- w184 stop-if-true
          n224 = local read "outcome"() -> (w189:u32)
          n225 = Not Equal?(x=w189, y=u32 0) -> (x != y?=w187:bool)
          n226 = case shown="True" w187 {
            tunnel: w194 -> [w197 w216]
            tunnel: w193 -> [w201 w211]
            tunnel: w192 -> [w199 w212]
            tunnel: [w200 w215] -> w191
            tunnel: [w198 w214] -> w183
            tunnel: [w196 w213] -> w190
            frame False {
              w196 = FALSE ("Boolean")
              n227 = Not Equal?(x=w196, y=w197) -> (x != y?=w195:bool)
              n228 = case shown="True" w195 {
                tunnel: w201 -> [w203 w209]
                tunnel: [w203 w208] -> w200
                tunnel: w199 -> [w202 w207]
                tunnel: [w202 w206] -> w198
                frame False {
                }
                frame True {
                  n229 = call "labjack.vi"("error out"=w207, "Boolean"=FALSE, "Handle Out"=w209) -> ("error out 2"=w206:errorcluster, "Boolean 2"=w204:bool, "Handle Out 2"=w208:i32)  [unwired: 6 in]
                  n230 = local write "Output"(w204) -> ()
                }
              }
            }
            frame True {
              n231 = local read "PWM"() -> (w213:bool)
              n232 = Not Equal?(x=w216, y=w213) -> (x != y?=w210:bool)
              n233 = case shown="True" w210 {
                tunnel: w211 -> [w218 w224]
                tunnel: w212 -> [w217 w223]
                tunnel: [w218 w222] -> w215
                tunnel: [w217 w221] -> w214
                frame False {
                }
                frame True {
                  n234 = local read "PWM"() -> (w220:bool)
                  n235 = call "labjack.vi"("error out"=w223, "Boolean"=w220, "Handle Out"=w224) -> ("error out 2"=w221:errorcluster, "Boolean 2"=w219:bool, "Handle Out 2"=w222:i32)  [unwired: 6 in]
                  n236 = local write "Output"(w219) -> ()
                }
              }
            }
          }
          n237 = Wait (ms)(milliseconds to wait=u32 5) -> ()  [unwired: 1 out]
          n238 = local read "Stop Program"() -> (w185:bool)
          n239 = Or(x=w183, y=w185) -> (x .or. y?=w184:bool)
        }
        n240 = Merge Errors(w100, w130, w172) -> (w99:errorcluster)
        n241 = Release Queue(queue=w111, error in (no error)=w99) -> (error out=w102:errorcluster)  [unwired: 1 in, 2 out]
        n242 = Release Notifier(notifier=w101, error in (no error)=w102) -> (error out=w98:errorcluster)  [unwired: 1 in, 2 out]
        n243 = VISA Write(VISA resource name=w121, write buffer="S", error in (no error)=w98) -> (VISA resource name out=w120:refnum<visa-resource-name>, error out=w122:errorcluster)  [unwired: 1 out]
        n244 = Close File(refnum=w129, error in=w122) -> (error out=w128:errorcluster)  [unwired: 1 out]
        n245 = call "rename_xml.vi"("error in"=w128, "xml"=w125, "csv"=w126) -> ("error out"=w127:errorcluster)  [unwired: 4 in]
        n246 = VISA Close(VISA resource name=w120, error in (no error)=w127) -> (error out=w153:errorcluster)
        n247 = call "labjack.vi"("error out"=w153, "Boolean"=FALSE, "Handle Out"=w148) -> ("error out 2"=w154:errorcluster, "Handle Out 2"=w152:i32)  [unwired: 6 in, 1 out]
        n248 = call "LJM_Close.vi"("error in"=w154, "Handle"=w152) -> ("error out"=w151:errorcluster)  [unwired: 9 in]
        "error out" <- w151
        n249 = call "LJM_ErrorToString.vi"("error in"=w151) -> ("String"=→"Error String":string)  [unwired: 10 in]
      }
    }
    n250 = local write "millisecond timer value 2"("millisecond timer value 2") -> ()
    n251 = Wait (ms)(milliseconds to wait=u32 5) -> ()  [unwired: 1 out]
    n252 = local read "Stop Program"() -> (w94:bool)
  }
  n253 = local read "deleted portion"() -> (→"deleted portion":u8[])
  n254 = local read "Output"() -> (→"Output":bool)
  n255 = local read "Sign"() -> (→"Sign":bool)
  n256 = local read "PWM"() -> (→"PWM":bool)
  n257 = local read "data"() -> (→"data":bool)
  n258 = local read "Read"() -> (→"Read":bool)
  n259 = flat-sequence {
    tunnel: w10 -> [w584]
    tunnel: [w584] -> w9
    tunnel: w9 -> [w585]
    frame #0 {
      n260 = Not(x=w584) -> (.not. x?=w583:bool)
      n261 = local write "Stop Program"(w583) -> ()
    }
    frame #1 {
      n262 = Stop(stop? (T)=w585) -> ()
    }
  }
  "Progress" <- 0.0 ("Slide")
  "Time" <- 0.0 ("Progress 2")
